vi "timestamps.vi"(1 "points recorded":i32=5, 2 "# of frames":i32=200 min=1 step=1, 3 "timestamps in":string[](array[string]), 4 "command":string) -> (0 "timestamps out":string[](array[string]))   [LabVIEW 2015]
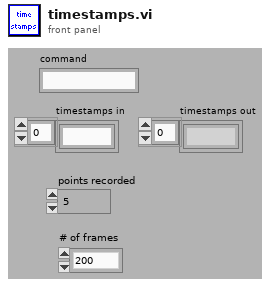
[diagram p1: front panel]
types:
  T1 = typedef "LVRectTypeDef.ctl" = cluster{"Left":i16, "Top":i16, "Right":i16, "Bottom":i16}
  T2 = cluster{"Xpixels":i32, "Vxminref":dbl, "Vxmaxref":dbl, "P":dbl, "Ypixels":i32, "Vyminref":dbl, "Vymaxref":dbl, "srate":sgl, "sAOxy":i32, "timeout":dbl, "type":string, "date":string, "time":string, "Colormap":u16, "Drawing Mode":u16, "Scanning Mode":u16, "square pixels":bool, "square matrix":bool, "Xpixels Img":i32, "Vx-min Img":dbl, "VX-max Img":dbl, "Ypixels Img":i32, "Vy-min Img":dbl, "Vy-max Img ":dbl, "Angle Img":dbl, "autoshutter":bool, "finite":bool, "cont":bool, "wavdet":bool, "measpoints":i32, "avpp":i32, "bufferAO":i32, "bufferAI":i32, "starttick":u32, "waveform":path, "Vx-ref":dbl, "Vy-ref":dbl, "refreshrate":dbl, "refreshbuffer":i32, "tt_cycles":i32, "motorref":refnum<k7>, "mirrorswitch":refnum<k7>, "sample mode":i32, "maxbufferAI":i32, "srateAODO":sgl, "bin":sgl, "Pel":sgl, "Angle draw":dbl, "srate Img":sgl, "ROIimg_plotbounds":T1, "auto OD":bool, "ODfilt":u16, "aAI":i32[], "aCI":i32[], "aAO":u32[], "aDO":u32[], "refwfsize":dbl, "Lifetime":bool, "Vz-Img":dbl, "Vz-ref":dbl, "Vz-reset":dbl, "AIoverride":bool}
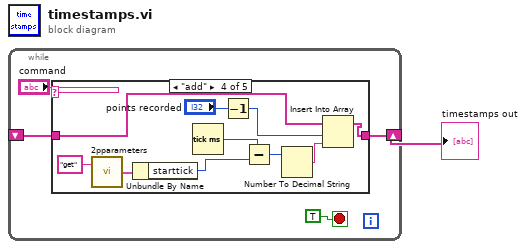
[diagram p0: block diagram]
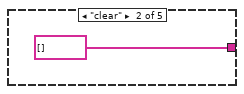
[diagram p3: hidden frame]
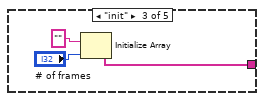
[diagram p4: hidden frame]
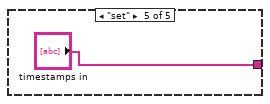
[diagram p5: hidden frame]
diagram:
  n1 = while {
    shift-right: [w3] -> w1
    shift-left: _ -> [w2]
    stop <- TRUE stop-if-true
    n2 = case shown="\"add\"" "command" {
      tunnel: [w6 string[] [] ("timestamps") w8 w12 "timestamps in"] -> w3
      tunnel: w2 -> [w6 _ _ w11 _]
      frame "get", Default {
      }
      frame "clear" {
      }
      frame "init" {
        n3 = Initialize Array("", "# of frames") -> (w8:string[])
      }
      frame "add" {
        n4 = call "2pparameters.vi"("command"="get") -> ("params out"=w15:T2)  [unwired: 1 in]
        n5 = Unbundle By Name(w15) -> ("starttick"=w14:u32)
        n6 = Tick Count (ms)() -> (millisecond timer value=w19:u32)
        n7 = Decrement(x="points recorded") -> (x-1=w13:i32)
        n8 = Subtract(x=w19, y=w14) -> (x-y=w18:u32)
        n9 = Number To Decimal String(number=w18) -> (decimal integer string=w17:string)  [unwired: 1 in]
        n10 = Insert Into Array(array=w11, index=w13, new element=w17) -> (w12:string[])
      }
      frame "set" {
      }
    }
  }
  "timestamps out" <- w1
